vi "Inficon Example.vi"(8 "Error In":errorcluster, 10 "Remote Port":u16=502, 11 "Remote IP Address":string="192.168.1.32") -> (0 "Error Out":errorcluster, 3 "Inficon Data Output":T1={"Gross Heating Value, Vol (Real, Dry)"=1067.4462890625, "Nitrogen Component Normalized Mole % (Dry)"=0.0, "Methane Component Normalized Mole % (Dry)"=92.87550354003906, "Carbon Dioxide Component Normalized Mole % (Dry)"=0.1941000074148178, "Ethane Component Normalized Mole % (Dry)"=6.454999923706055, "Propane Component Normalized Mole % (Dry)"=0.3865000009536743, "i-Pentane Component Normalized Mole % (Dry)"=0.007799999788403511, "i-Butane Component Normalized Mole % (Dry)"=0.03880000114440918, "n-Butane Component Normalized Mole % (Dry)"=0.03819999843835831, "n-Pentane Component Normalized Mole % (Dry)"=0.004100000020116568, "Hexane Component Normalized Mole % (Dry)"=0.0, "Heptane Component Normalized Mole % (Dry)"=0.0, "Gross Wobbe Index, Real(Dry)"=1385.8905029296875, "Relative Density, Real(Dry)"=0.5932452082633972, "Propylene Component Normalized Mole % (Dry)"=0.0, "C4 Olefins Component Normalized Mole % (Dry)"=0.0, "Water Component Normalized Mole % (Dry)"=0.0})   [LabVIEW 2019]
uses:
  Type Definitions/Inficon Data.ctl
  <vilib>/NI/Modbus Library/API/Master/Modbus Master.lvclass
  <vilib>/NI/Modbus Library/API/Wrapper/Create TCP Master.vi
  <vilib>/NI/Modbus Library/API/Wrapper/API Main.lvlib
panel:
  out "Text Array":string[][](array[string])
  in  "address":string
  in  "Inficon Data Input":T1
  # "Natural Gas"
  # "Propane"
  # "Natural Gas"
  # "Propane"
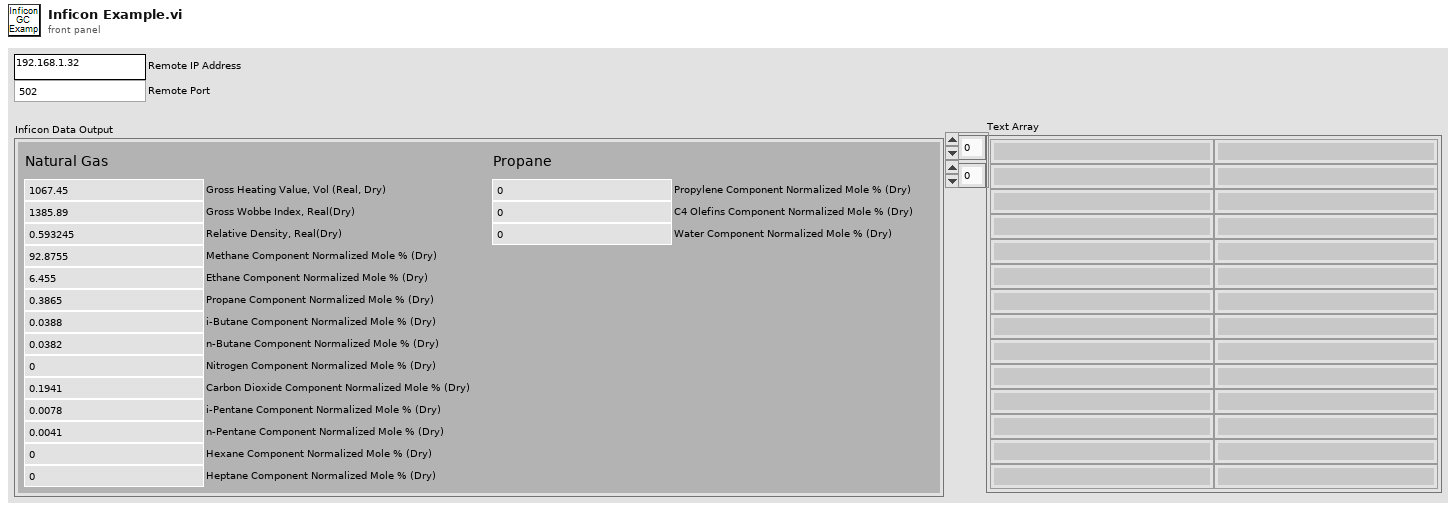
[diagram p1: front panel]
types:
  T1 = typedef "Inficon Data.ctl" = cluster{"Gross Heating Value, Vol (Real, Dry)":dbl, "Nitrogen Component Normalized Mole % (Dry)":dbl, "Methane Component Normalized Mole % (Dry)":dbl, "Carbon Dioxide Component Normalized Mole % (Dry)":dbl, "Ethane Component Normalized Mole % (Dry)":dbl, "Propane Component Normalized Mole % (Dry)":dbl, "i-Pentane Component Normalized Mole % (Dry)":dbl, "i-Butane Component Normalized Mole % (Dry)":dbl, "n-Butane Component Normalized Mole % (Dry)":dbl, "n-Pentane Component Normalized Mole % (Dry)":dbl, "Hexane Component Normalized Mole % (Dry)":dbl, "Heptane Component Normalized Mole % (Dry)":dbl, "Gross Wobbe Index, Real(Dry)":dbl, "Relative Density, Real(Dry)":dbl, "Propylene Component Normalized Mole % (Dry)":dbl, "C4 Olefins Component Normalized Mole % (Dry)":dbl, "Water Component Normalized Mole % (Dry)":dbl}
  T2 = enum32{"invalid app kind", "Development System", "Run Time System", "Student Edition", "Embedded LabVIEW", "Evaluation", "Custom"}
  T3 = enum32{"Invalid", "Standard", "Closed", "Hidden", "Minimized", "Maximized"}
  T4 = cluster{"Core":cluster{"Current VI Reference":refnum<vi>, "Close Panel on Exit?":bool}, "Remote IP Address":string, "Remote Port":u16, "TCP master instance":refnum<class "Modbus Master.lvclass">, "Inficon Data Input":T1}
  T5 = cluster{"Current VI Reference":refnum<vi>, "Close Panel on Exit?":bool}
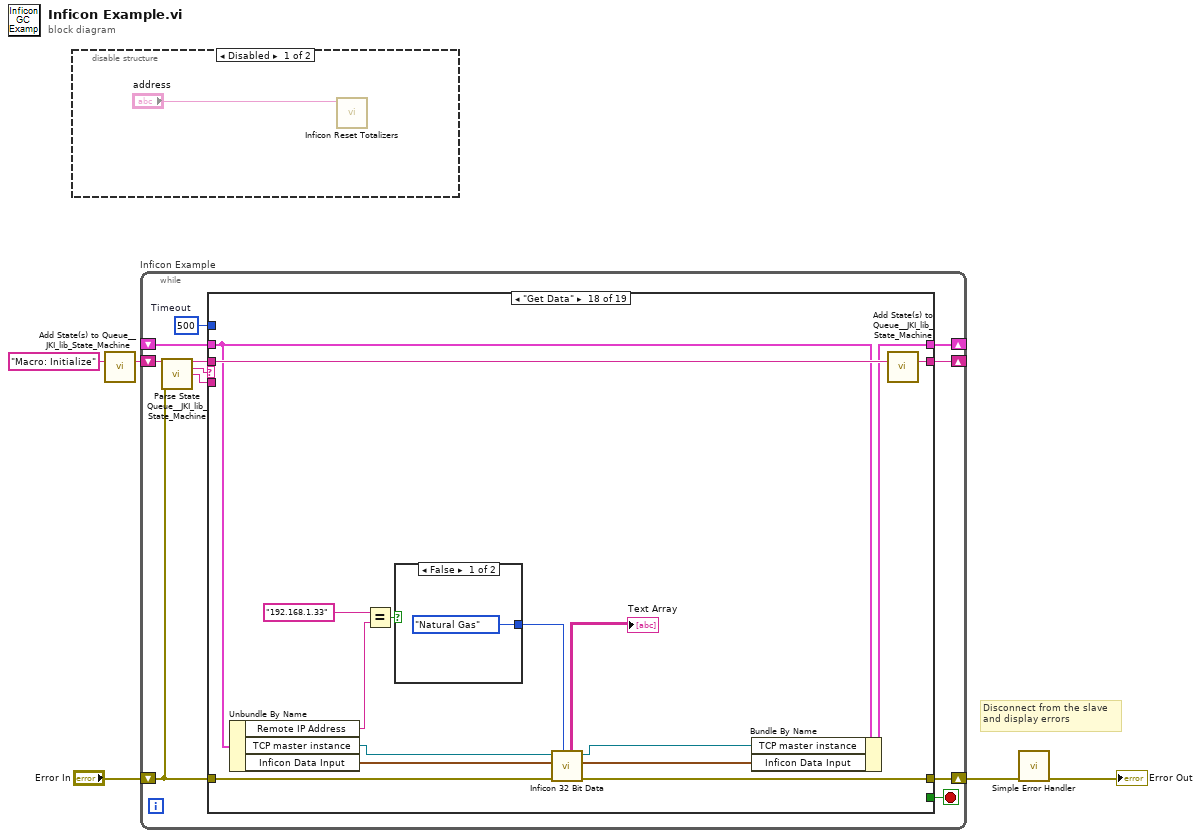
[diagram p0: block diagram]
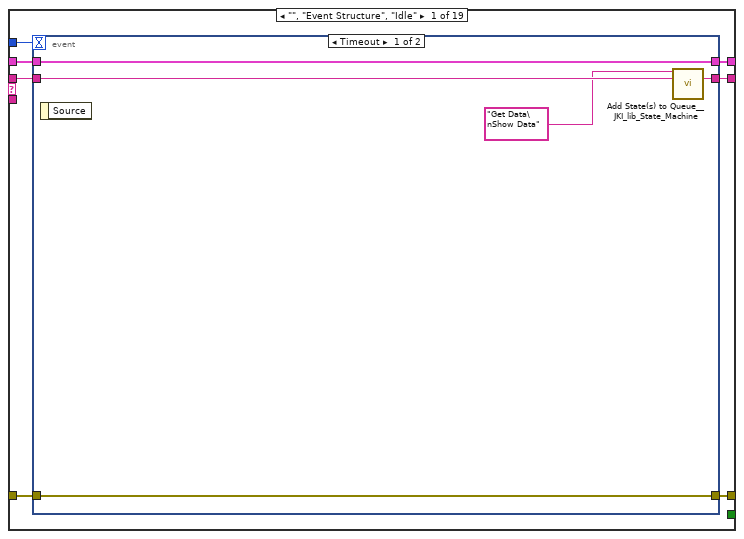
[diagram p3: hidden frame]
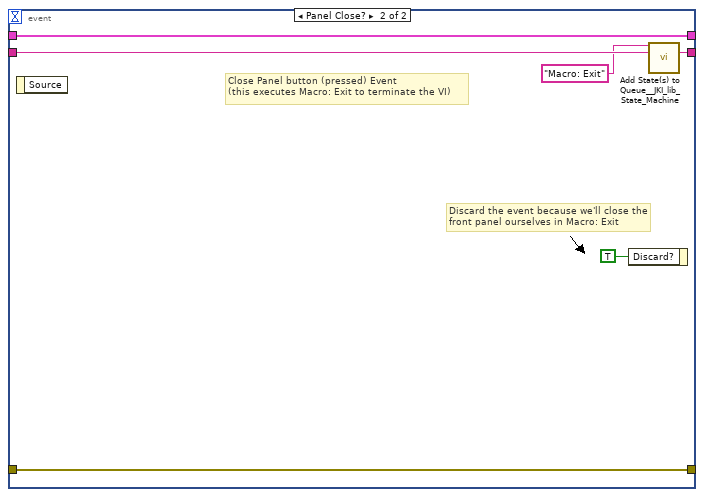
[diagram p4: hidden frame]
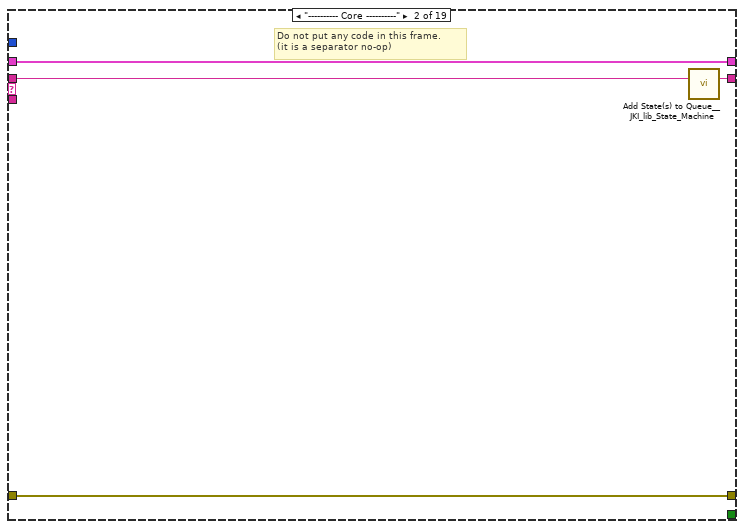
[diagram p5: hidden frame]
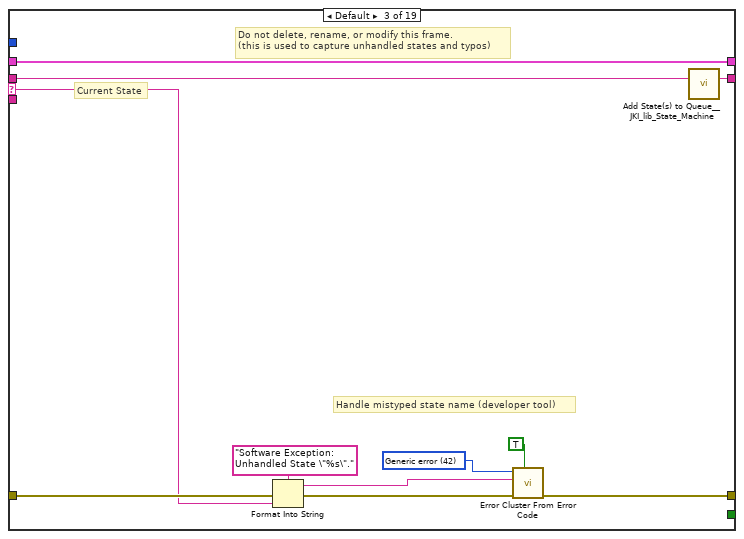
[diagram p6: hidden frame]
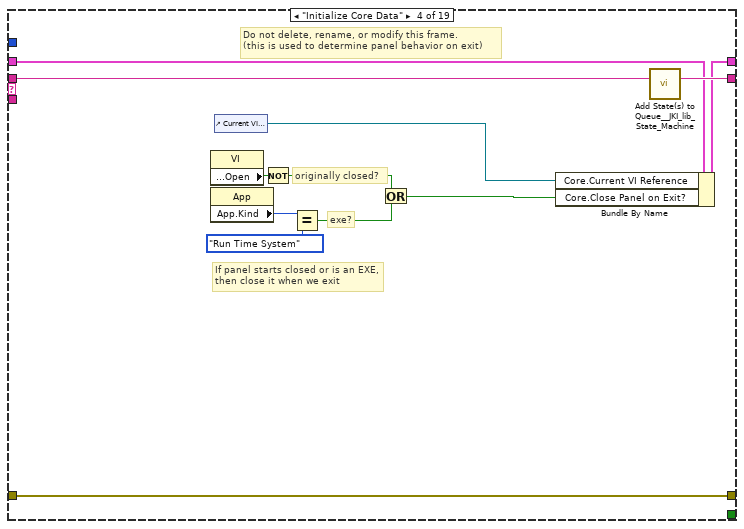
[diagram p7: hidden frame]
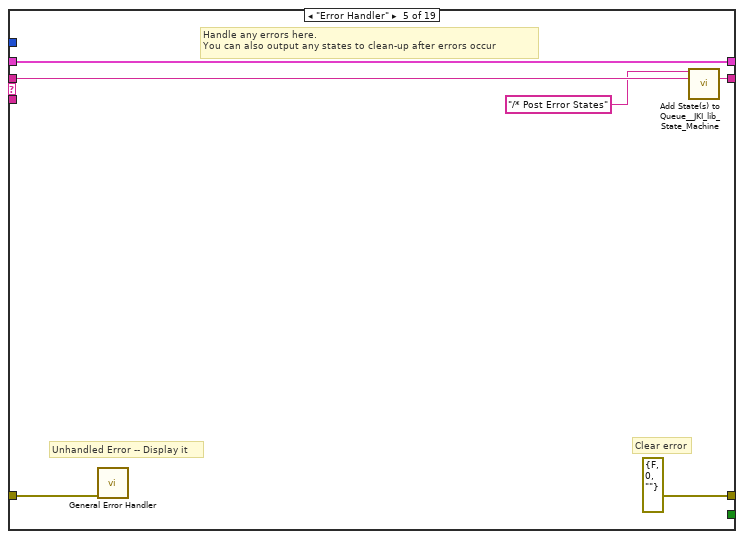
[diagram p8: hidden frame]
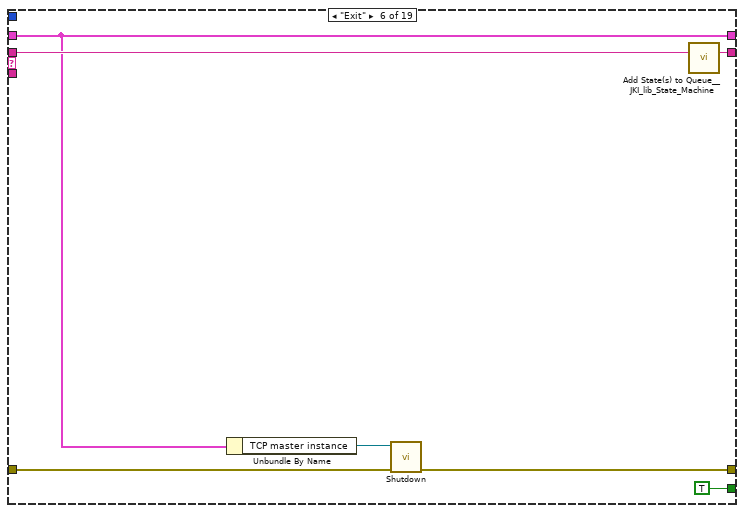
[diagram p9: hidden frame]
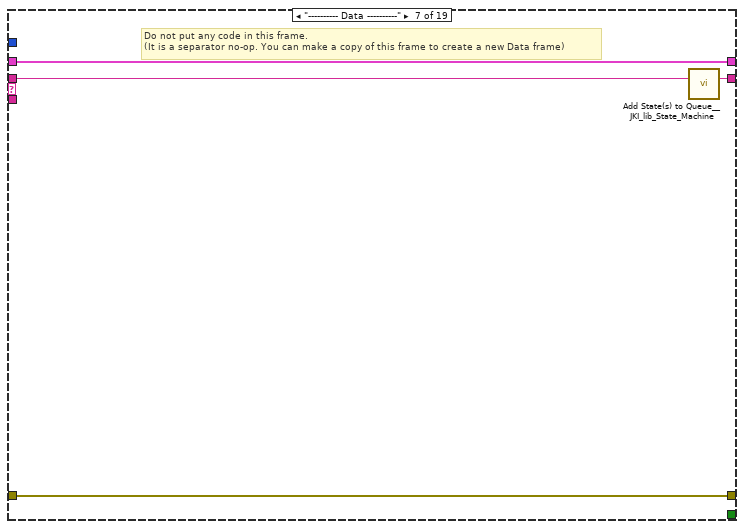
[diagram p10: hidden frame]
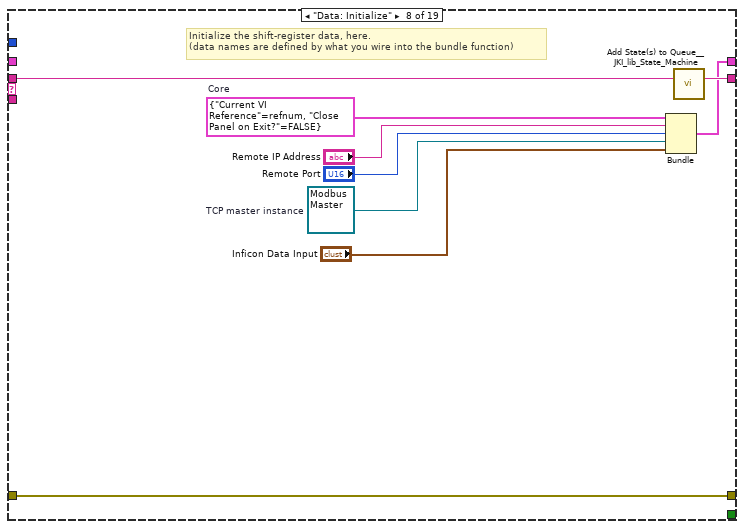
[diagram p11: hidden frame]
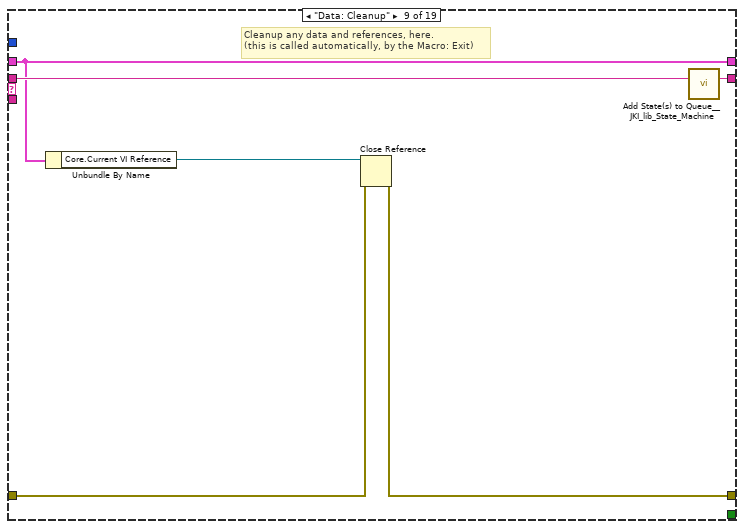
[diagram p12: hidden frame]
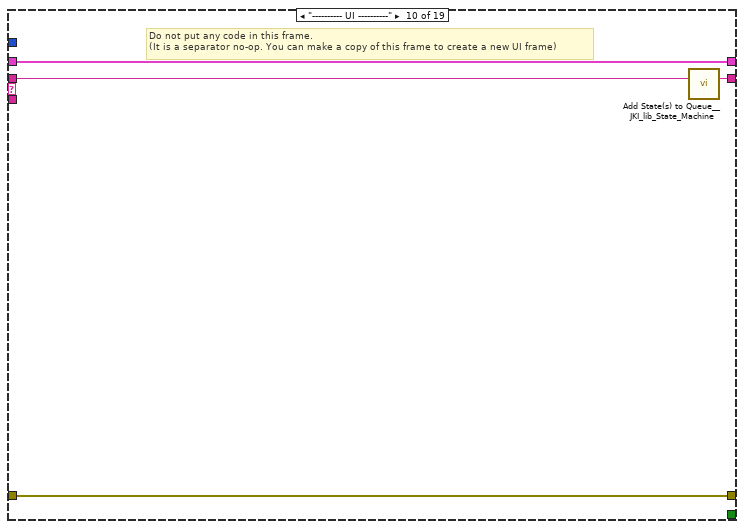
[diagram p13: hidden frame]
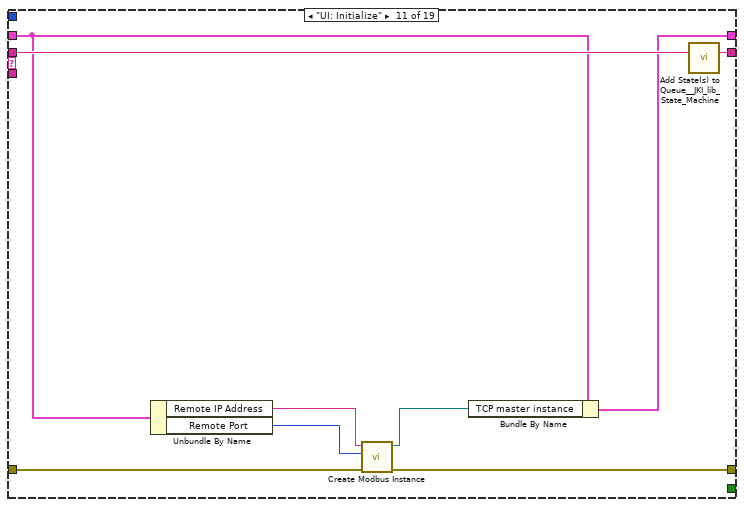
[diagram p14: hidden frame]
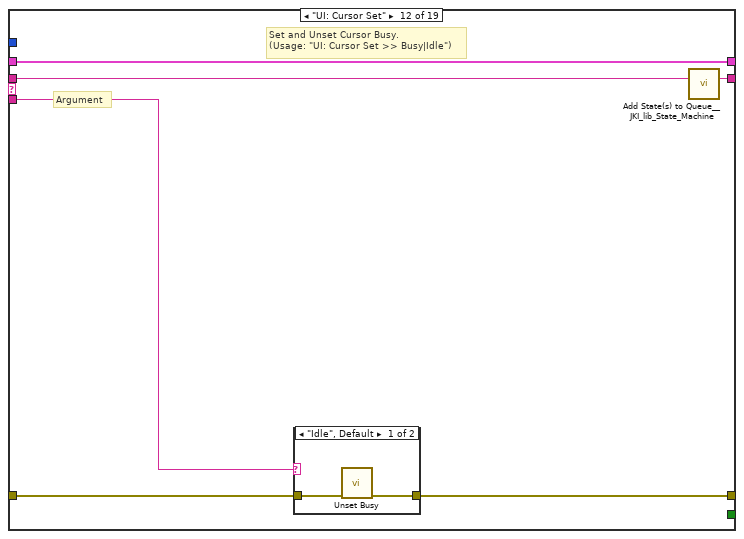
[diagram p15: hidden frame]
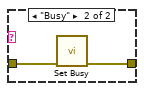
[diagram p16: hidden frame]
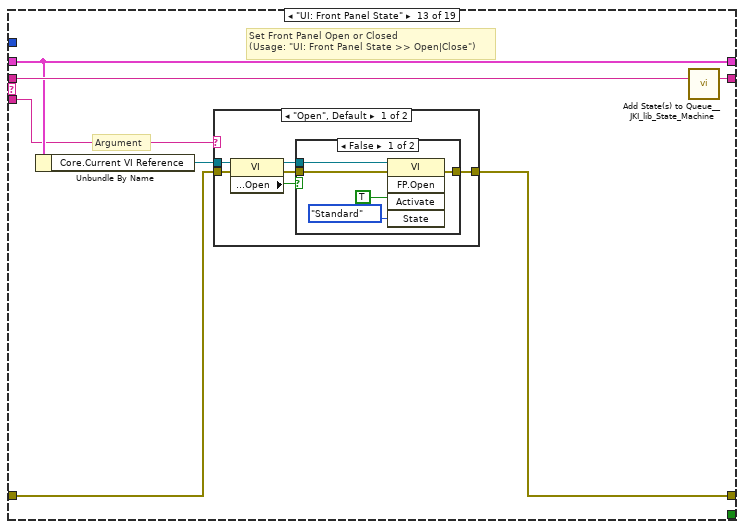
[diagram p17: hidden frame]
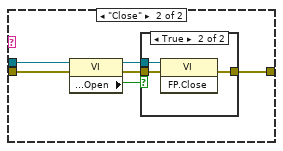
[diagram p19: hidden frame]
diagram:
  # "Disconnect from the slave\nand display errors"
  n1 = disable-structure shown="Disabled" {
    frame Disabled {
      n2 = call "Inficon Reset Totalizers.vi"("address"="address") -> ()  [unwired: 10 in, 1 out]
    }
    frame Enabled {
    }
  }
  n3 = call <vilib>:"Add State(s) to Queue__JKI_lib_State_Machine.vi"("State(s) in (\"\")"="Macro: Initialize") -> ("States Out"=w5:string)  [unwired: 14 in]
  n4 = while "Inficon Example" {
    shift-right: [w10] -> _
    shift-left: _ -> [w9]
    shift-right: [w13] -> w2
    shift-left: "Error In" -> [w7]
    shift-right: [w12] -> _
    shift-left: w5 -> [w14]
    stop <- w11 stop-if-true
    w8 = 500  # Timeout
    n5 = call <vilib>:"Parse State Queue__JKI_lib_State_Machine.vi"("State Queue"=w14, "Error In (no error)"=w7) -> ("Remaining States"=w16:string, "Current State"=w17:string, "Arguments"=w15:string)  [unwired: 11 in]
    n6 = case shown="\"Get Data\"" w17 {
      selector: w17 -> [_ _ w40 _ _ _ _ _ _ _ _ _ _ _ _ _ _ _ _]
      tunnel: w16 -> [w24 w39 w44 w62 w68 w75 w79 w88 w94 w98 w107 w113 w124 w150 w155 w165 w169 w184 w191]
      tunnel: w15 -> [_ _ _ _ _ _ _ _ _ _ _ w108 w118 _ _ _ _ _ _]
      tunnel: w9 -> [w22 w36 w42 w53 w65 w70 w76 _ w89 w95 w101 w111 w120 w147 w152 w162 w166 w181 w188]
      tunnel: [w21 w37 w46 w59 errorcluster {"status"=FALSE, "code"=0, "source"=""} ("error out") w71 w77 w85 w90 w96 w104 w109 w121 w148 w153 w163 w167 w182 w189] -> w13
      tunnel: w7 -> [w20 w37 w45 w59 w64 w72 w77 w85 w91 w96 w105 w110 w122 w148 w153 w163 w167 w177 w189]
      tunnel: [w23 w38 w43 w61 w67 w74 w78 w87 w93 w97 w106 w112 w123 w149 w154 w164 w168 w183 w190] -> w12
      tunnel: [_ _ _ _ _ TRUE _ _ _ _ _ _ _ _ _ _ _ _ _] -> w11
      tunnel: [w19 w36 w42 w60 w65 w70 w76 w86 w89 w95 w100 w111 w120 w147 w152 w162 w166 w180 w188] -> w10
      tunnel: w8 -> [w18 _ _ _ _ _ _ _ _ _ _ _ _ _ _ _ _ _ _]
      frame "", "Event Structure", "Idle" {
        n7 = event shown="[0] Timeout" {
          selector: _ -> [_ _]
          dyn-events: _ -> [_ _]
          timeout: w18 -> [_ _]
          tunnel: w24 -> [w29 w35]
          tunnel: [w28 w34] -> w23
          tunnel: w22 -> [w26 w32]
          tunnel: [w27 w33] -> w21
          tunnel: w20 -> [w27 w33]
          tunnel: [w26 w32] -> w19
          event Timeout {
            n8 = event-data() -> ()  [unwired: 1 in, 1 out]
            n9 = call <vilib>:"Add State(s) to Queue__JKI_lib_State_Machine.vi"("State(s) in Front (\"\")"="Get Data\nShow Data" ("State(s) in Front (\"\")"), "State(s) in (\"\")"=w29) -> ("States Out"=w28:string)  [unwired: 13 in]
          }
          event Panel Close? {
            # "Discard the event because we'll close the front panel ourselves in Macro: Exit"
            # "Close Panel button (pressed) Event\n(this executes Macro: Exit to terminate the VI)"
            n10 = event-data() -> ()  [unwired: 1 in, 1 out]
            n11 = event-data("Discard?"=TRUE) -> ()  [unwired: 1 in, 1 out]
            n12 = call <vilib>:"Add State(s) to Queue__JKI_lib_State_Machine.vi"("State(s) in Front (\"\")"="Macro: Exit", "State(s) in (\"\")"=w35) -> ("States Out"=w34:string)  [unwired: 13 in]
          }
        }
      }
      frame "---------- Core ----------" {
        # "Do not put any code in this frame.\n(it is a separator no-op)"
        n13 = call <vilib>:"Add State(s) to Queue__JKI_lib_State_Machine.vi"("State(s) in (\"\")"=w39) -> ("States Out"=w38:string)  [unwired: 14 in]
      }
      frame Default {
        w49 = 42 items=["No error", "Argument error", "Memory is full", "Out of zone", "End of file", "File already open", "Generic file I/O error", "File not found", "File permission error", "Disk is full", "Duplicate path", "Too many files open", "System feature not enabled", "Resource file not found", "Cannot add resource", "Resource not found", "Image not found", "Image memory error", "Pen does not exist", "Config type invalid", "Config token not found", "Config parse error", "Config memory error", "Bad external code format", "Bad external code offset", "External code not present", "Null window", "Destroy window error", "Null menu", "Print aborted", "Bad print record", "Print driver error", "Windows error during printing", "Memory error during printing", "Print dialog error", "Generic print error", "Invalid device refnum", "Device not found", "Device parameter error", "Device unit error", "Cannot open device", "Device call aborted", "Generic error", "Cancelled by user", "Object ID too low", "Object ID too high", "Object not in heap", "Unknown heap", "Unknown object (invalid DefProc)", "Unknown object (DefProc not in table)", "Message out of range", "Invalid (null) method", "Unknown message", "Manager call not supported", "Bad address", "Network operation in progress", "Network operation timed out", "Connection is busy", "Network attribute not supported", "Network error", "Address in use", "System out of memory", "Connection aborted", "Connection refused", "Not connected", "Already connected", "Connection closed", "Initialization error (interapplication manager)", "Bad occurrence", "Wait on unbound occurrence handler", "Occurrence queue overflow", "Datalog type conflict", "Unused", "Unrecognized type (interapplication manager)", "Memory corrupt", "Failed to make temporary DLL", "Old CIN version", "Drag socket not found", "Failed to load drop-object", "Failed to register OLE object", "Failed to release OLE object", "Format specifier type mismatch", "Unknown format specifier", "Too few format specifiers", "Too many format specifiers", "Scan failed", "Newer CIN version", "Error converting to variant", "Runtime menu error", "Password tampered", "Variant attribute not found", "Incompatible variant data type", "Event data is not available", "Event Store is not present", "Occurrence is not found", "Event Queue is not created", "Event info is not available", "Refnum passed is NULL", "Error retrieving Class GUID", "Error retrieving CoClass GUID", "Error retrieving TypeLib GUID.", "Bad built application magic bytes.", "Specific driver is different from the specific driver associated with the Logical Name.", "There is no session opened to the class driver.", "Max Error", "MAX - Error with config objects", "MAX - Error loading configuration", "MAX - Group not supported"]
        # "Current State"
        # "Do not delete, rename, or modify this frame.\n(this is used to capture unhandled states and typos)"
        # "Handle mistyped state name (developer tool)"
        n14 = Format Into String(format string="Software Exception: Unhandled State \"%s\"." ("message"), error in=w45, w40) -> (resulting string=w48:string, error out=w47:errorcluster)  [unwired: 1 in]
        n15 = call <vilib>:"Error Cluster From Error Code.vi"("show call chain? (False)"=TRUE, "error in (no error)"=w47, "error message (\"\")"=w48, "error code (0)"=w49) -> ("error out"=w46:errorcluster)  [unwired: 5 in]
        n16 = call <vilib>:"Add State(s) to Queue__JKI_lib_State_Machine.vi"("State(s) in (\"\")"=w44) -> ("States Out"=w43:string)  [unwired: 14 in]
      }
      frame "Initialize Core Data" {
        # "Do not delete, rename, or modify this frame.\n(this is used to determine panel behavior on exit)"
        # "originally closed?"
        # "exe?"
        # "If panel starts closed or is an EXE, then close it when we exit"
        n17 = property class="VI"() -> ("Front Panel.Open"=w58:bool)  [unwired: 2 in, 2 out]
        n18 = property class="App"() -> ("App.Kind"=w57:T2)  [unwired: 2 in, 2 out]
        n19 = control-ref of="Current VI Reference"() -> (w51:refnum<vi>)
        n20 = Not(x=w58) -> (.not. x?=w55:bool)
        n21 = Equal?(x=w57, y=T2."Run Time System" ("Application:Kind")) -> (x = y?=w54:bool)
        n22 = Or(x=w55, y=w54) -> (x .or. y?=w52:bool)
        n23 = Bundle By Name(cluster=w53, "Core.Current VI Reference"=w51, "Core.Close Panel on Exit?"=w52) -> (w60:T4)
        n24 = call <vilib>:"Add State(s) to Queue__JKI_lib_State_Machine.vi"("State(s) in (\"\")"=w62) -> ("States Out"=w61:string)  [unwired: 14 in]
      }
      frame "Error Handler" {
        # "Unhandled Error -- Display it"
        # "Handle any errors here.\nYou can also output any states to clean-up after errors occur"
        # "Clear error"
        n25 = call <vilib>:"General Error Handler.vi"("error in (no error)"=w64) -> ()  [unwired: 10 in, 5 out]
        n26 = call <vilib>:"Add State(s) to Queue__JKI_lib_State_Machine.vi"("State(s) in Front (\"\")"="/* Post Error States", "State(s) in (\"\")"=w68) -> ("States Out"=w67:string)  [unwired: 13 in]
      }
      frame "Exit" {
        n27 = Unbundle By Name(w70) -> ("TCP master instance"=w69:refnum<class "Modbus Master.lvclass">)
        n28 = call-dynamic "Shutdown.vi"("error in"=w72, "Modbus master in"=w69) -> ("error out"=w71:errorcluster)  [unwired: 9 in]
        n29 = call <vilib>:"Add State(s) to Queue__JKI_lib_State_Machine.vi"("State(s) in (\"\")"=w75) -> ("States Out"=w74:string)  [unwired: 14 in]
      }
      frame "---------- Data ----------" {
        # "Do not put any code in this frame.\n(It is a separator no-op. You can make a copy of this frame to create a new Data frame)"
        n30 = call <vilib>:"Add State(s) to Queue__JKI_lib_State_Machine.vi"("State(s) in (\"\")"=w79) -> ("States Out"=w78:string)  [unwired: 14 in]
      }
      frame "Data: Initialize" {
        w81 = refnum<class "Modbus Master.lvclass"> refnum  # TCP master instance
        w84 = T5 {"Current VI Reference"=refnum, "Close Panel on Exit?"=FALSE}  # Core
        # "Initialize the shift-register data, here.\n(data names are defined by what you wire into the bundle function)"
        n31 = Bundle("Core"=w84, "Remote IP Address"="Remote IP Address", "Remote Port"="Remote Port", "TCP master instance"=w81, "Inficon Data Input"="Inficon Data Input") -> (w86:T4)  [unwired: 1 in]
        n32 = call <vilib>:"Add State(s) to Queue__JKI_lib_State_Machine.vi"("State(s) in (\"\")"=w88) -> ("States Out"=w87:string)  [unwired: 14 in]
      }
      frame "Data: Cleanup" {
        # "Cleanup any data and references, here.\n(this is called automatically, by the Macro: Exit)"
        n33 = Unbundle By Name(w89) -> ("Core.Current VI Reference"=w92:refnum<vi>)
        n34 = Close Reference(reference=w92, error in (no error)=w91) -> (error out=w90:errorcluster)
        n35 = call <vilib>:"Add State(s) to Queue__JKI_lib_State_Machine.vi"("State(s) in (\"\")"=w94) -> ("States Out"=w93:string)  [unwired: 14 in]
      }
      frame "---------- UI ----------" {
        # "Do not put any code in this frame.\n(It is a separator no-op. You can make a copy of this frame to create a new UI frame)"
        n36 = call <vilib>:"Add State(s) to Queue__JKI_lib_State_Machine.vi"("State(s) in (\"\")"=w98) -> ("States Out"=w97:string)  [unwired: 14 in]
      }
      frame "UI: Initialize" {
        n37 = Unbundle By Name(w101) -> ("Remote IP Address"=w103:string, "Remote Port"=w102:u16)
        n38 = call-poly <vilib>:"Create Modbus Instance.vi"("error in"=w105, "port (502)"=w102, "address"=w103) -> ("error out"=w104:errorcluster, "TCP master instance"=w99:refnum<class "Modbus Master.lvclass">)  [unwired: 7 in]
        n39 = Bundle By Name(cluster=w101, "TCP master instance"=w99) -> (w100:T4)
        n40 = call <vilib>:"Add State(s) to Queue__JKI_lib_State_Machine.vi"("State(s) in (\"\")"=w107) -> ("States Out"=w106:string)  [unwired: 14 in]
      }
      frame "UI: Cursor Set" {
        # "Argument"
        # "Set and Unset Cursor Busy.\n(Usage: \"UI: Cursor Set >> Busy|Idle\")"
        n41 = case shown="\"Idle\", Default" w108 {
          tunnel: w110 -> [w115 w117]
          tunnel: [w114 w116] -> w109
          frame "Idle", Default {
            n42 = call <vilib>:"Unset Busy.vi"("error in (no error)"=w115) -> ("error out"=w114:errorcluster)  [unwired: 10 in]
          }
          frame "Busy" {
            n43 = call <vilib>:"Set Busy.vi"("error in (no error)"=w117) -> ("error out"=w116:errorcluster)  [unwired: 9 in, 1 out]
          }
        }
        n44 = call <vilib>:"Add State(s) to Queue__JKI_lib_State_Machine.vi"("State(s) in (\"\")"=w113) -> ("States Out"=w112:string)  [unwired: 14 in]
      }
      frame "UI: Front Panel State" {
        # "Argument"
        # "Set Front Panel Open or Closed\n(Usage: \"UI: Front Panel State >> Open|Close\")"
        n45 = Unbundle By Name(w120) -> ("Core.Current VI Reference"=w119:refnum<vi>)
        n46 = case shown="\"Open\", Default" w118 {
          tunnel: w122 -> [w128 w141]
          tunnel: [w130 w142] -> w121
          tunnel: w119 -> [w129 w139]
          frame "Open", Default {
            n47 = property class="VI"(reference=w129, error in=w128) -> (reference out=w126:refnum<vi>, error out=w127:errorcluster, "Front Panel.Open"=w125:bool)
            n48 = case shown="False" w125 {
              tunnel: [w133 w136] -> w130
              tunnel: w127 -> [w132 w136]
              tunnel: w126 -> [w131 _]
              frame False {
                n49 = invoke class="VI" method="FP.Open"(reference=w131, error in=w132, "Activate"=TRUE, "State"=T3."Standard") -> (error out=w133:errorcluster)  [unwired: 1 in, 4 out]
              }
              frame True {
              }
            }
          }
          frame "Close" {
            n50 = property class="VI"(reference=w139, error in=w141) -> (reference out=w138:refnum<vi>, error out=w140:errorcluster, "Front Panel.Open"=w137:bool)
            n51 = case shown="True" w137 {
              tunnel: [w143 w146] -> w142
              tunnel: w140 -> [w143 w145]
              tunnel: w138 -> [_ w144]
              frame False {
              }
              frame True {
                n52 = invoke class="VI" method="FP.Close"(reference=w144, error in=w145) -> (error out=w146:errorcluster)  [unwired: 1 in, 2 out]
              }
            }
          }
        }
        n53 = call <vilib>:"Add State(s) to Queue__JKI_lib_State_Machine.vi"("State(s) in (\"\")"=w124) -> ("States Out"=w123:string)  [unwired: 14 in]
      }
      frame "---------- Macro ----------" {
        # "Do not put any code in this frame.\n(It is a separator no-op. You can make a copy of this frame to create a new Macro frame)"
        n54 = call <vilib>:"Add State(s) to Queue__JKI_lib_State_Machine.vi"("State(s) in (\"\")"=w150) -> ("States Out"=w149:string)  [unwired: 14 in]
      }
      frame "Macro: Initialize" {
        w151 = "Data: Initialize\nInitialize Core Data\nUI: Initialize\nUI: Front Panel State >> Open"  # Data: Initialize Initialize Core Data UI: Initialize UI: Front Panel State >> Open
        # "Initialization Macro\n(This is called once, when the VI starts)"
        n55 = call <vilib>:"Add State(s) to Queue__JKI_lib_State_Machine.vi"("State(s) in Front (\"\")"=w151, "State(s) in (\"\")"=w155) -> ("States Out"=w154:string)  [unwired: 13 in]
      }
      frame "Macro: Exit" {
        # "Exit Macro\n(This is called once, when the VI exits)"
        n56 = Unbundle By Name(w162) -> ("Core.Close Panel on Exit?"=w161:bool)
        n57 = Select(t="UI: Front Panel State >> Close", s=w161, f="") -> (s? t:f=w158:string)
        n58 = call <vilib>:"Add State(s) to Queue__JKI_lib_State_Machine.vi"("State(s) in (\"\")"=w158, "State(s) at Back (\"\")"="Data: Cleanup\nExit") -> ("States Out"=w156:string)  [unwired: 13 in]
        n59 = call <vilib>:"Add State(s) to Queue__JKI_lib_State_Machine.vi"("State(s) in Front (\"\")"=w156, "State(s) in (\"\")"=w165) -> ("States Out"=w164:string)  [unwired: 13 in]
      }
      frame "---------- New Category ----------" {
        # "Template Separator\n(You can make a copy of, or modify, this frame)"
        n60 = call <vilib>:"Add State(s) to Queue__JKI_lib_State_Machine.vi"("State(s) in (\"\")"=w169) -> ("States Out"=w168:string)  [unwired: 14 in]
      }
      frame "Get Data" {
        n61 = Unbundle By Name(w181) -> ("Remote IP Address"=w174:string, "TCP master instance"=w176:refnum<class "Modbus Master.lvclass">, "Inficon Data Input"=w175:T1)
        n62 = Equal?(x="192.168.1.33", y=w174) -> (x = y?=w172:bool)
        n63 = case shown="False" w172 {
          tunnel: [enum16{"Natural Gas", "Propane Gas"}."Natural Gas" ("Gas Type") enum16{"Natural Gas", "Propane Gas"}."Propane Gas" ("Gas Type")] -> w171
          frame False {
          }
          frame True {
          }
        }
        n64 = call "Inficon 32 Bit Data.vi"("Gas Type"=w171, "Error In"=w177, "Inficon Data Input"=w175, "Modbus master in"=w176) -> ("Error Out"=w182:errorcluster, "Inficon Data Output"=w178:T1, "Modbus master out"=w179:refnum<class "Modbus Master.lvclass">, "Text Array"=→"Text Array":string[][])  [unwired: 4 in]
        n65 = Bundle By Name(cluster=w181, "TCP master instance"=w179, "Inficon Data Input"=w178) -> (w180:T4)
        n66 = call <vilib>:"Add State(s) to Queue__JKI_lib_State_Machine.vi"("State(s) in (\"\")"=w184) -> ("States Out"=w183:string)  [unwired: 14 in]
      }
      frame "Show Data" {
        n67 = Unbundle By Name(w188) -> ("Inficon Data Input"=→"Inficon Data Output":T1)
        n68 = call <vilib>:"Add State(s) to Queue__JKI_lib_State_Machine.vi"("State(s) in (\"\")"=w191) -> ("States Out"=w190:string)  [unwired: 14 in]
      }
    }
  }
  n69 = call <vilib>:"Simple Error Handler.vi"("error in (no error)"=w2) -> ("error out"=→"Error Out":errorcluster)  [unwired: 1 in, 7 out]
